vi "Exit.vi"(8 "error in (no error)":errorcluster, 10 "Variant":variant) -> (0 "error out":errorcluster)   [LabVIEW 2020, in "COnfiguration Database.lvlib"]
doc: "Send Stop Message to the Queue."
uses:
  COnfiguration Database.lvlib
  Private Controls/Message Cluster.ctl
  Private Controls/Message enum.ctl
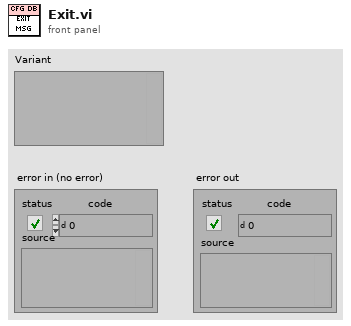
[diagram p1: front panel]
types:
  T1 = typedef "COnfiguration Database.lvlib/Message Cluster.ctl" = cluster{"Message":T2, "Data":variant}
  T2 = typedef "COnfiguration Database.lvlib/Message enum.ctl" = enum16{"Initialize", "Update DB", "Search DB", "Error", "Exit"}
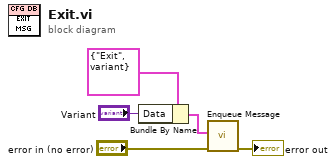
[diagram p0: block diagram]
diagram:
  n1 = Bundle By Name(cluster=T1 {"Message"=enum."Exit", "Data"=variant} ("Message Cluster"), "Data"="Variant") -> (w1:T1)
  n2 = call "Enqueue Message.vi"("error in (no error)"="error in (no error)", "Element"=w1) -> ("error out"=→"error out":errorcluster)  [unwired: 9 in]
